vi "Duplicate Disabled Frame Target.vi"(11 "Input":bool[](array[boolean])) -> (3 "Any?":bool)   [LabVIEW 2017, in "Tests.lvlib" / "Toolkit.lvlib"]
uses:
  Toolkit.lvlib
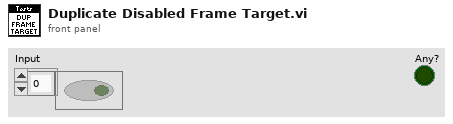
[diagram p1: front panel]
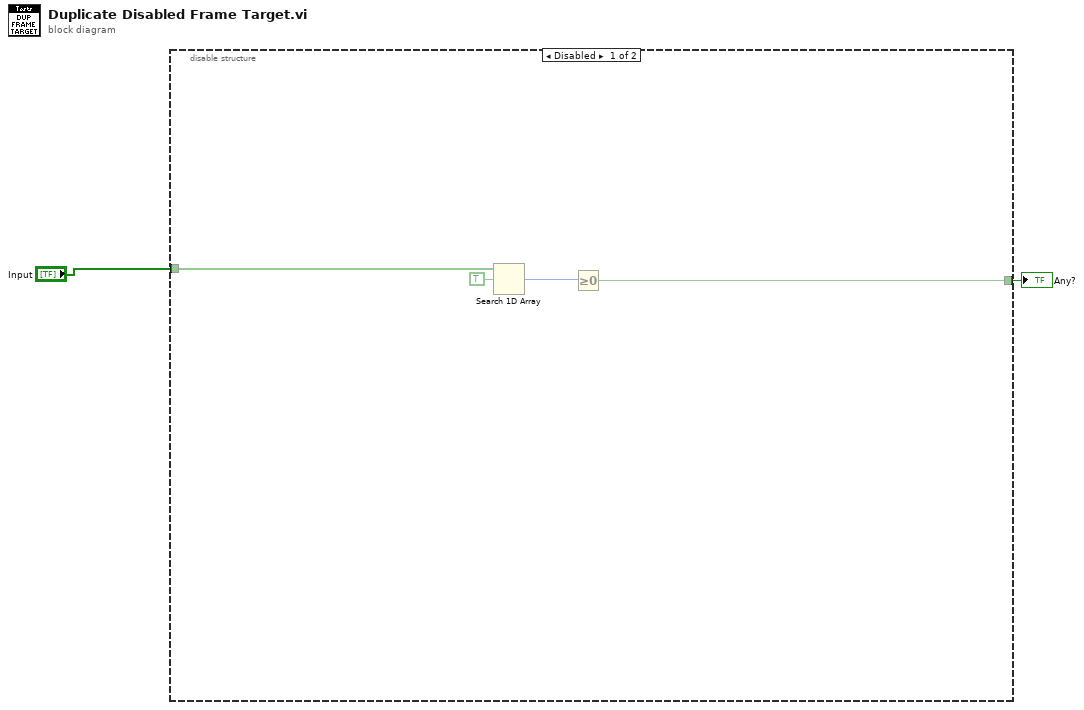
[diagram p0: block diagram]
diagram:
  n1 = disable-structure shown="Disabled" {
    disable-tunnel: "Input" -> [w6 _]
    disable-tunnel: [w3 _] -> w1
    frame Disabled {
      n2 = Search 1D Array(1D array=w6, element=TRUE) -> (index of element=w4:i32)  [unwired: 1 in]
      n3 = Greater Or Equal To 0?(x=w4) -> (x >= 0?=w3:bool)
    }
    frame Enabled {
    }
  }
  "Any?" <- w1
